vi "LinTableSubVI.vi"(2 "Step":dbl, 3 "Final":dbl, 4 "Initial":dbl) -> (1 "Array":dbl[](array[numeric]))   [LabVIEW 2017]
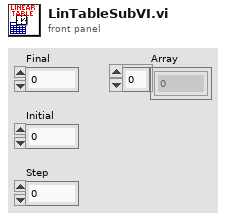
[diagram p1: front panel]
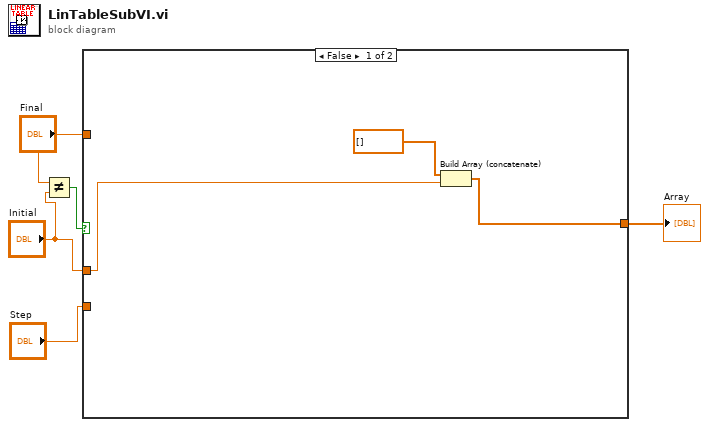
[diagram p0: block diagram]
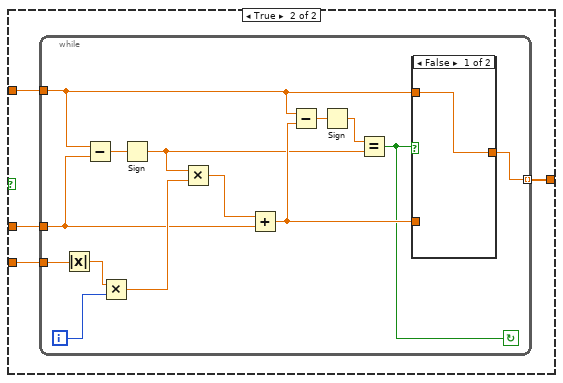
[diagram p2: hidden frame]
diagram:
  n1 = Not Equal?(x="Final", y="Initial") -> (x != y?=w2:bool)
  n2 = case shown="False" w2 {
    tunnel: "Initial" -> [w6 w12]
    tunnel: "Step" -> [_ w11]
    tunnel: "Final" -> [_ w10]
    tunnel: [w7 w9] -> w4
    frame False {
      n3 = Build Array (concatenate)(dbl[] [], w6) -> (w7:dbl[])
    }
    frame True {
      n4 = while {
        tunnel: [w22] -> w9 mode=indexing
        tunnel: w10 -> [w16]
        tunnel: w11 -> [w13]
        tunnel: w12 -> [w17]
        i -> [w24]
        stop <- w15 continue-if-true
        n5 = Absolute Value(x=w13) -> (abs(x)=w14:dbl)
        n6 = Subtract(x=w16, y=w17) -> (x-y=w26:dbl)
        n7 = Multiply(x=w14, y=w24) -> (x*y=w23:dbl)
        n8 = Sign(1:w26) -> (0:w18:dbl)
        n9 = Multiply(x=w18, y=w23) -> (x*y=w21:dbl)
        n10 = Add(x=w21, y=w17) -> (x+y=w20:dbl)
        n11 = Subtract(x=w16, y=w20) -> (x-y=w25:dbl)
        n12 = Sign(1:w25) -> (0:w19:dbl)
        n13 = Equal?(x=w19, y=w18) -> (x = y?=w15:bool)
        n14 = case shown="False" w15 {
          tunnel: [w27 w28] -> w22
          tunnel: w20 -> [_ w28]
          tunnel: w16 -> [w27 _]
          frame False {
          }
          frame True {
          }
        }
      }
    }
  }
  "Array" <- w4
